vi "_Register.vi"(8 "Error In":errorcluster, 10 "Listener ID":string, 11 "Listeners In":refnum<queue>[](array[refnum])) -> (0 "Error Out":errorcluster, 3 "Listeners Out":refnum<queue>[](array[refnum]))   [LabVIEW 2014, in "LV-Logger.lvlib"]
uses:
  LV-Logger.lvlib
  Public/Controls/Message.ctl
  Public/Controls/Level.ctl
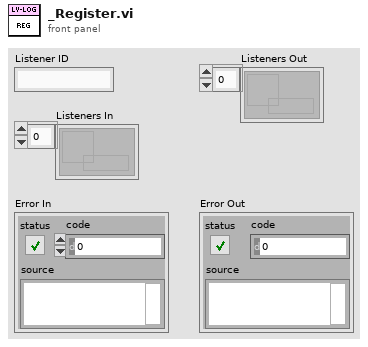
[diagram p1: front panel]
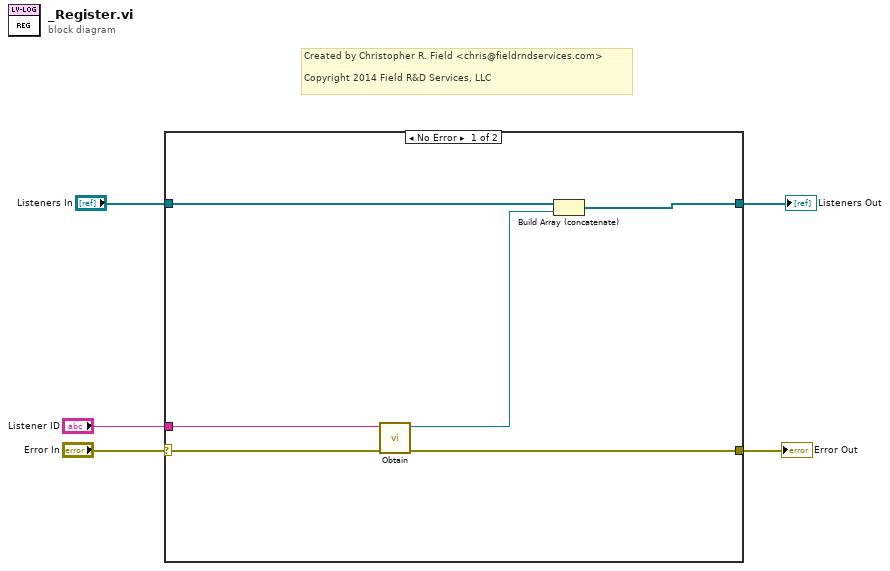
[diagram p0: block diagram]
diagram:
  # "Created by Christopher R. Field <chris@fieldrndservices.com>\n\nCopyright 2014 Field R&D Services, LLC"
  n1 = case shown="No Error" "Error In" {
    selector: "Error In" -> [w6 w13]
    tunnel: "Listener ID" -> [w9 _]
    tunnel: "Listeners In" -> [w11 w12]
    tunnel: [w10 w12] -> w3
    tunnel: [w7 w13] -> w2
    frame No Error {
      n2 = call "Obtain.vi"("Error In"=w6, "Listener ID"=w9) -> ("Error Out"=w7:errorcluster, "Listener"=w8:refnum<queue>)  [unwired: 8 in]
      n3 = Build Array (concatenate)(w11, w8) -> (w10:refnum<queue>[])
    }
    frame Error {
    }
  }
  "Listeners Out" <- w3
  "Error Out" <- w2
